vi "DT_Triangle Manager_Get Adj_by Edge.vi"(8 "point idx 2":i32, 9 "point idx 1":i32, 10 "triangle":i32, 11 "Triangles":i32[][](array[numeric])) -> (2 "adj triangle":i32)   [LabVIEW 2020, in "NI_AAL_Geometry.lvlib"]
uses:
  <vilib>/Analysis/NI_AAL_Geometry.lvlib
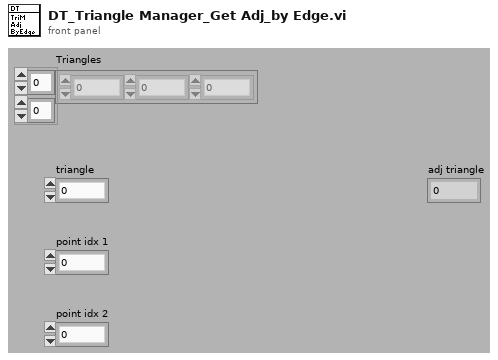
[diagram p1: front panel]
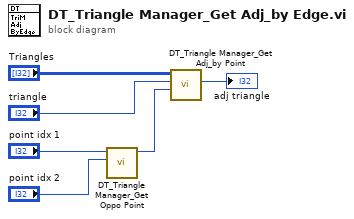
[diagram p0: block diagram]
diagram:
  n1 = call <vilib>:"DT_Triangle Manager_Get Oppo Point.vi"("point idx 2"="point idx 2", "point idx 1"="point idx 1") -> ("oppo point idx"=w6:i32)  [unwired: 9 out]
  n2 = call <vilib>:"DT_Triangle Manager_Get Adj_by Point.vi"("point idx"=w6, "triangle"="triangle", "Triangles In"="Triangles") -> ("adj triangle"=→"adj triangle":i32)  [unwired: 8 out]
